vi "ControlPlot.vi"(6 "MatchBallY":dbl, 7 "MatchBallX":dbl, 8 "D2 Y COM":dbl, 9 "D2 X COM":dbl, 10 "D1Y COM":dbl, 11 "D1 X COM 2":dbl) -> (1 "XY Graph 3":cluster{dbl[], dbl[]}(graph), 2 "XY Graph 2":cluster{dbl[], dbl[]}(graph), 3 "XY Graph":cluster{dbl[], dbl[]}(graph))   [LabVIEW 2014]
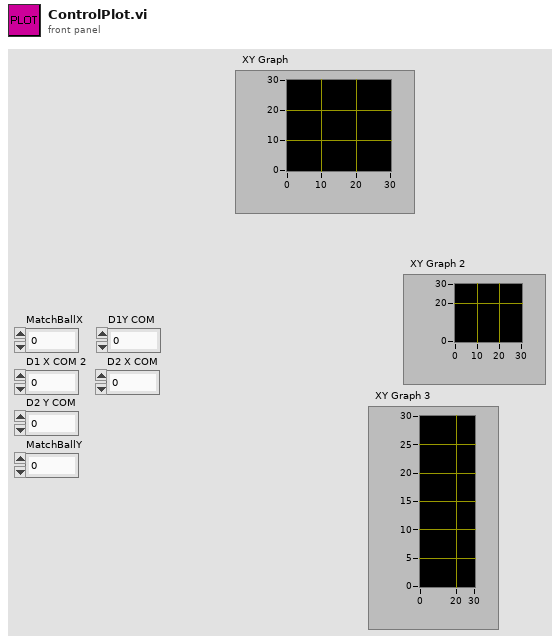
[diagram p1: front panel]
types:
  T1 = cluster{"m":dbl, "MatchBallX":dbl, "type":dbl, "MatchBallY":dbl}
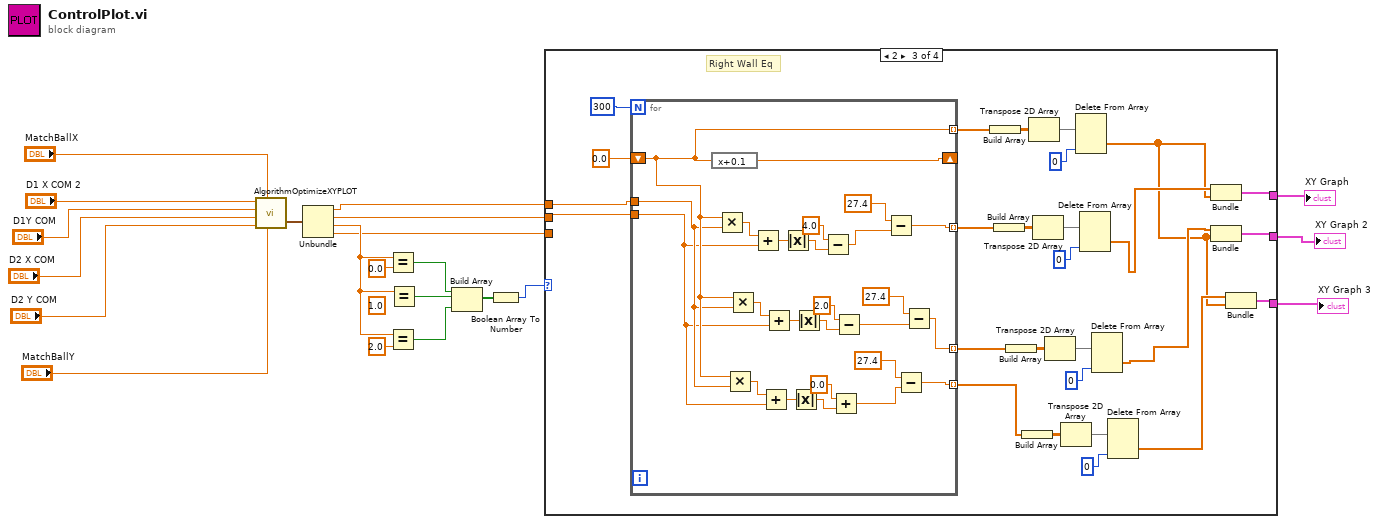
[diagram p0: block diagram]
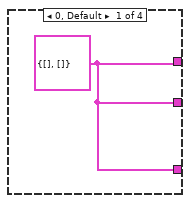
[diagram p2: hidden frame]
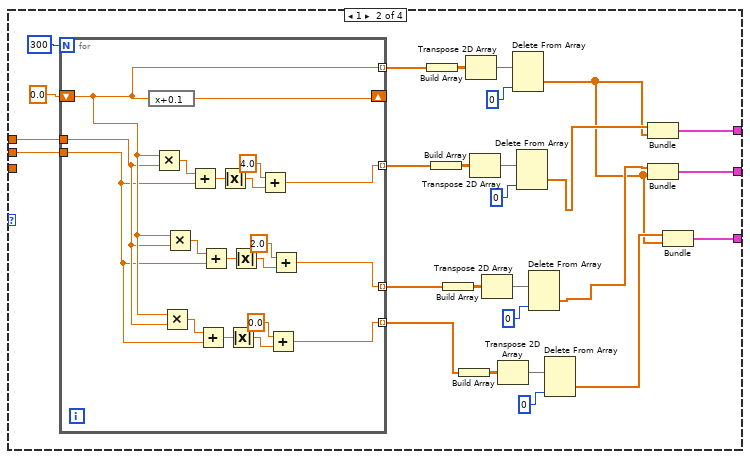
[diagram p3: hidden frame]
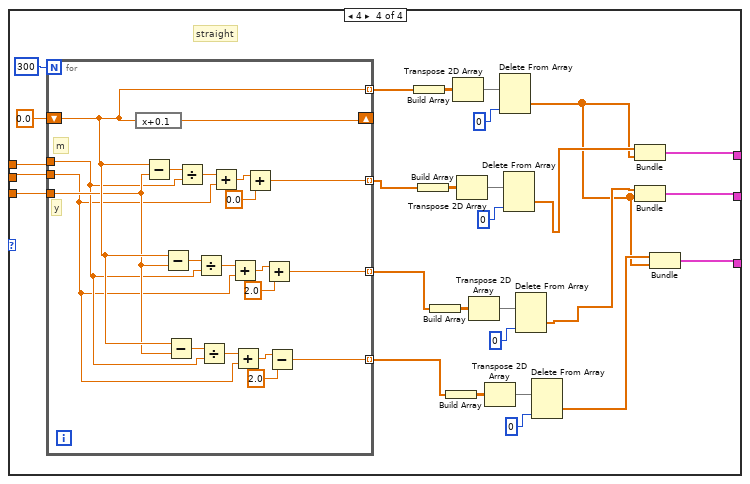
[diagram p4: hidden frame]
diagram:
  (unwired) 1.0
  n1 = call "AlgorithmOptimizeXYPLOT.vi"("MatchBallY"="MatchBallY", "MatchBallX"="MatchBallX", "D2 Y COM"="D2 Y COM", "D2 X COM"="D2 X COM", "D1Y COM"="D1Y COM", "D1 X COM 2"="D1 X COM 2") -> ("Plot"=w15:T1)  [unwired: 1 out]
  n2 = Unbundle(w15) -> ("m"=w6:dbl, "MatchBallX"=w5:dbl, "type"=w11:dbl, "MatchBallY"=w4:dbl)
  n3 = Equal?(x=w11, y=0.0) -> (x = y?=w12:bool)
  n4 = Equal?(x=w11, y=2.0) -> (x = y?=w8:bool)
  n5 = Equal?(x=w11) -> (x = y?=w9:bool)  [unwired: 1 in]
  n6 = Build Array(w12, w9, w8) -> (w13:bool[])
  n7 = Boolean Array To Number(Boolean array=w13) -> (number=w7:u32)
  n8 = case shown="2" w7 {
    tunnel: w6 -> [_ w27 w73 w128]
    tunnel: w5 -> [_ w26 w72 w127]
    tunnel: w4 -> [_ _ _ w129]
    tunnel: [w22 w25 w71 w123] -> w3
    tunnel: [w22 w24 w70 w122] -> w2
    tunnel: [w22 w23 w69 w121] -> w1
    frame 0, Default {
      w22 = cluster{dbl[], dbl[]} {[], []}
    }
    frame 1 {
      n9 = for {
        N: 300 -> [_]
        shift-right: [w68] -> _
        shift-left: 0.0 -> [w53]
        tunnel: [w53] -> w47 mode=indexing
        tunnel: [w63] -> w40 mode=indexing
        tunnel: [w58] -> w34 mode=indexing
        tunnel: [w50] -> w30 mode=indexing
        tunnel: w27 -> [w52]
        tunnel: w26 -> [w51]
        n10 = expression code="x+0.1"(w53) -> (w68:dbl)
        n11 = Multiply(x=w53, y=w52) -> (x*y=w67:dbl)
        n12 = Multiply(x=w53, y=w52) -> (x*y=w54:dbl)
        n13 = Multiply(x=w53, y=w52) -> (x*y=w62:dbl)
        n14 = Add(x=w67, y=w51) -> (x+y=w66:dbl)
        n15 = Add(x=w54, y=w51) -> (x+y=w55:dbl)
        n16 = Add(x=w62, y=w51) -> (x+y=w61:dbl)
        n17 = Absolute Value(x=w66) -> (abs(x)=w65:dbl)
        n18 = Absolute Value(x=w55) -> (abs(x)=w56:dbl)
        n19 = Absolute Value(x=w61) -> (abs(x)=w60:dbl)
        n20 = Add(x=4.0, y=w65) -> (x+y=w63:dbl)
        n21 = Add(x=0.0, y=w56) -> (x+y=w50:dbl)
        n22 = Add(x=2.0, y=w60) -> (x+y=w58:dbl)
      }
      n23 = Build Array(w47) -> (w46:dbl[][])
      n24 = Build Array(w40) -> (w41:dbl[][])
      n25 = Build Array(w34) -> (w37:dbl[][])
      n26 = Build Array(w30) -> (w33:dbl[][])
      n27 = Transpose 2D Array(2D array=w46) -> (transposed array=w45:dbl[][])
      n28 = Transpose 2D Array(2D array=w41) -> (transposed array=w42:dbl[][])
      n29 = Transpose 2D Array(2D array=w37) -> (transposed array=w38:dbl[][])
      n30 = Transpose 2D Array(2D array=w33) -> (transposed array=w32:dbl[][])
      n31 = Delete From Array(array=w45, index (col)=0 ("disabled index (col)")) -> (deleted portion=w28:dbl[])  [unwired: 2 in, 1 out]
      n32 = Delete From Array(array=w42, index (col)=0 ("disabled index (col)")) -> (deleted portion=w35:dbl[])  [unwired: 2 in, 1 out]
      n33 = Delete From Array(array=w38, index (col)=0 ("disabled index (col)")) -> (deleted portion=w36:dbl[])  [unwired: 2 in, 1 out]
      n34 = Delete From Array(array=w32, index (col)=0 ("disabled index (col)")) -> (deleted portion=w29:dbl[])  [unwired: 2 in, 1 out]
      n35 = Bundle(w35, w28) -> (w25:cluster{dbl[], dbl[]})  [unwired: 1 in]
      n36 = Bundle(w36, w28) -> (w24:cluster{dbl[], dbl[]})  [unwired: 1 in]
      n37 = Bundle(w29, w28) -> (w23:cluster{dbl[], dbl[]})  [unwired: 1 in]
    }
    frame 2 {
      # "Right Wall Eq"
      n38 = for {
        N: 300 -> [_]
        shift-right: [w120] -> _
        shift-left: 0.0 -> [w107]
        tunnel: [w107] -> w93 mode=indexing
        tunnel: [w104] -> w86 mode=indexing
        tunnel: [w96] -> w80 mode=indexing
        tunnel: [w97] -> w76 mode=indexing
        tunnel: w73 -> [w106]
        tunnel: w72 -> [w105]
        n39 = expression code="x+0.1"(w107) -> (w120:dbl)
        n40 = Multiply(x=w107, y=w106) -> (x*y=w119:dbl)
        n41 = Multiply(x=w107, y=w106) -> (x*y=w108:dbl)
        n42 = Multiply(x=w107, y=w106) -> (x*y=w115:dbl)
        n43 = Add(x=w119, y=w105) -> (x+y=w118:dbl)
        n44 = Add(x=w108, y=w105) -> (x+y=w109:dbl)
        n45 = Add(x=w115, y=w105) -> (x+y=w114:dbl)
        n46 = Absolute Value(x=w118) -> (abs(x)=w117:dbl)
        n47 = Absolute Value(x=w109) -> (abs(x)=w110:dbl)
        n48 = Absolute Value(x=w114) -> (abs(x)=w113:dbl)
        n49 = Subtract(x=4.0, y=w117) -> (x-y=w102:dbl)
        n50 = Add(x=0.0, y=w110) -> (x+y=w98:dbl)
        n51 = Subtract(x=2.0, y=w113) -> (x-y=w99:dbl)
        n52 = Subtract(x=27.4, y=w102) -> (x-y=w104:dbl)
        n53 = Subtract(x=27.4, y=w98) -> (x-y=w97:dbl)
        n54 = Subtract(x=27.4, y=w99) -> (x-y=w96:dbl)
      }
      n55 = Build Array(w93) -> (w92:dbl[][])
      n56 = Build Array(w86) -> (w87:dbl[][])
      n57 = Build Array(w80) -> (w83:dbl[][])
      n58 = Build Array(w76) -> (w79:dbl[][])
      n59 = Transpose 2D Array(2D array=w92) -> (transposed array=w91:dbl[][])
      n60 = Transpose 2D Array(2D array=w87) -> (transposed array=w88:dbl[][])
      n61 = Transpose 2D Array(2D array=w83) -> (transposed array=w84:dbl[][])
      n62 = Transpose 2D Array(2D array=w79) -> (transposed array=w78:dbl[][])
      n63 = Delete From Array(array=w91, index (col)=0 ("disabled index (col)")) -> (deleted portion=w74:dbl[])  [unwired: 2 in, 1 out]
      n64 = Delete From Array(array=w88, index (col)=0 ("disabled index (col)")) -> (deleted portion=w81:dbl[])  [unwired: 2 in, 1 out]
      n65 = Delete From Array(array=w84, index (col)=0 ("disabled index (col)")) -> (deleted portion=w82:dbl[])  [unwired: 2 in, 1 out]
      n66 = Delete From Array(array=w78, index (col)=0 ("disabled index (col)")) -> (deleted portion=w75:dbl[])  [unwired: 2 in, 1 out]
      n67 = Bundle(w81, w74) -> (w71:cluster{dbl[], dbl[]})  [unwired: 1 in]
      n68 = Bundle(w82, w74) -> (w70:cluster{dbl[], dbl[]})  [unwired: 1 in]
      n69 = Bundle(w75, w74) -> (w69:cluster{dbl[], dbl[]})  [unwired: 1 in]
    }
    frame 4 {
      # "straight"
      n70 = for {
        N: 300 -> [_]
        shift-right: [w168] -> _
        shift-left: 0.0 -> [w154]
        tunnel: [w154] -> w146 mode=indexing
        tunnel: w128 -> [w152]
        tunnel: w127 -> [w151]
        tunnel: w129 -> [w153]
        tunnel: [w163] -> w126 mode=indexing
        tunnel: [w150] -> w125 mode=indexing
        tunnel: [w149] -> w124 mode=indexing
        # "y"
        # "m"
        n71 = expression code="x+0.1"(w154) -> (w168:dbl)
        n72 = Subtract(x=w154, y=w153) -> (x-y=w167:dbl)
        n73 = Subtract(x=w154, y=w153) -> (x-y=w159:dbl)
        n74 = Subtract(x=w154, y=w153) -> (x-y=w158:dbl)
        n75 = Divide(x=w167, y=w152) -> (x/y=w166:dbl)
        n76 = Divide(x=w159, y=w152) -> (x/y=w160:dbl)
        n77 = Divide(x=w158, y=w152) -> (x/y=w157:dbl)
        n78 = Add(x=w166, y=w151) -> (x+y=w165:dbl)
        n79 = Add(x=w160, y=w151) -> (x+y=w161:dbl)
        n80 = Add(x=w157, y=w151) -> (x+y=w156:dbl)
        n81 = Add(x=w165, y=0.0) -> (x+y=w163:dbl)
        n82 = Add(x=w161, y=2.0) -> (x+y=w150:dbl)
        n83 = Subtract(x=w156, y=2.0) -> (x-y=w149:dbl)
      }
      n84 = Build Array(w146) -> (w145:dbl[][])
      n85 = Build Array(w126) -> (w140:dbl[][])
      n86 = Build Array(w125) -> (w137:dbl[][])
      n87 = Build Array(w124) -> (w134:dbl[][])
      n88 = Transpose 2D Array(2D array=w145) -> (transposed array=w144:dbl[][])
      n89 = Transpose 2D Array(2D array=w140) -> (transposed array=w141:dbl[][])
      n90 = Transpose 2D Array(2D array=w137) -> (transposed array=w138:dbl[][])
      n91 = Transpose 2D Array(2D array=w134) -> (transposed array=w133:dbl[][])
      n92 = Delete From Array(array=w144, index (col)=0 ("disabled index (col)")) -> (deleted portion=w130:dbl[])  [unwired: 2 in, 1 out]
      n93 = Delete From Array(array=w141, index (col)=0 ("disabled index (col)")) -> (deleted portion=w135:dbl[])  [unwired: 2 in, 1 out]
      n94 = Delete From Array(array=w138, index (col)=0 ("disabled index (col)")) -> (deleted portion=w136:dbl[])  [unwired: 2 in, 1 out]
      n95 = Delete From Array(array=w133, index (col)=0 ("disabled index (col)")) -> (deleted portion=w131:dbl[])  [unwired: 2 in, 1 out]
      n96 = Bundle(w135, w130) -> (w123:cluster{dbl[], dbl[]})  [unwired: 1 in]
      n97 = Bundle(w136, w130) -> (w122:cluster{dbl[], dbl[]})  [unwired: 1 in]
      n98 = Bundle(w131, w130) -> (w121:cluster{dbl[], dbl[]})  [unwired: 1 in]
    }
  }
  "XY Graph" <- w3
  "XY Graph 2" <- w2
  "XY Graph 3" <- w1
